vi "SSC DCPower Configure Output Enabled And Connected.vi"(0 "DCPower SSC in":T1[](array[typedef]), 5 "Output Enabled And Connected":bool, 11 "error in":errorcluster) -> (4 "DCPower SSC out":T1[](array[typedef]), 15 "error out":errorcluster)   [LabVIEW 2020]
doc: "This VI configures output enabled and connected on the channels.\n\nT - Enable and then connect\nF - Disconnect and then disable"
uses:
  SSC DCPower.ctl
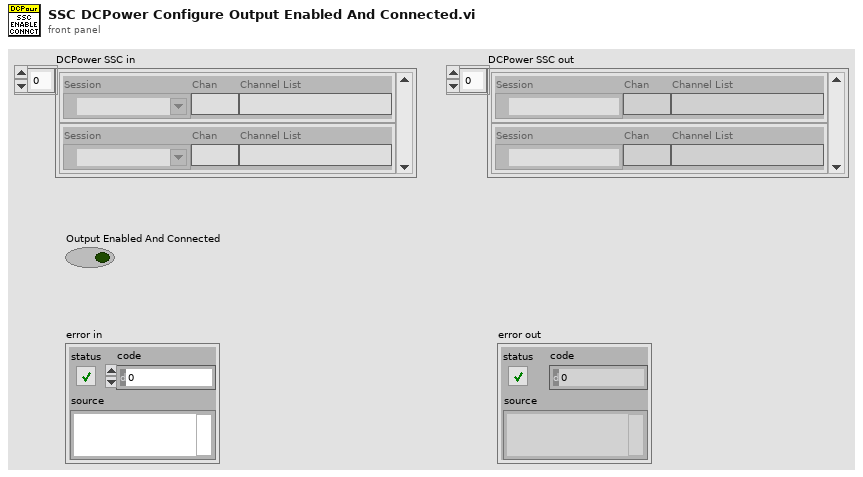
[diagram p1: front panel]
types:
  T1 = typedef "SSC DCPower.ctl" = cluster{"Session":refnum<k15>, "Chan":string, "Channel List":string}
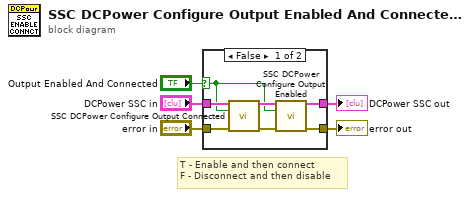
[diagram p0: block diagram]
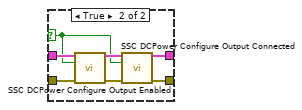
[diagram p2: hidden frame]
diagram:
  # "T - Enable and then connect\nF - Disconnect and then disable"
  n1 = case shown="False" "Output Enabled And Connected" {
    selector: "Output Enabled And Connected" -> [w6 w13]
    tunnel: "error in" -> [w12 w19]
    tunnel: [w9 w16] -> w4
    tunnel: "DCPower SSC in" -> [w10 w17]
    tunnel: [w7 w14] -> w2
    frame False {
      n2 = call "SSC DCPower Configure Output Connected.vi"("DCPower SSC in"=w10, "Output Connected"=w6, "error in"=w12) -> ("DCPower SSC out"=w8:T1[], "error out"=w11:errorcluster)  [unwired: 11 in]
      n3 = call "SSC DCPower Configure Output Enabled.vi"("DCPower SSC in"=w8, "Output Enabled"=w6, "error in"=w11) -> ("DCPower SSC out"=w7:T1[], "error out"=w9:errorcluster)  [unwired: 11 in]
    }
    frame True {
      n4 = call "SSC DCPower Configure Output Enabled.vi"("DCPower SSC in"=w17, "Output Enabled"=w13, "error in"=w19) -> ("DCPower SSC out"=w15:T1[], "error out"=w18:errorcluster)  [unwired: 11 in]
      n5 = call "SSC DCPower Configure Output Connected.vi"("DCPower SSC in"=w15, "Output Connected"=w13, "error in"=w18) -> ("DCPower SSC out"=w14:T1[], "error out"=w16:errorcluster)  [unwired: 11 in]
    }
  }
  "error out" <- w4
  "DCPower SSC out" <- w2
